vi "initialize python session.vi"(8 "error in (no error)":errorcluster, 11 "Save Image in":refnum<class "Save Image.lvclass">) -> (0 "error out":errorcluster, 3 "Save Image out":refnum<class "Save Image.lvclass">)   [LabVIEW 2018, in "Save Image.lvclass"]
doc: "Initialize the Python Toolkit"
uses:
  Save Image.lvclass
  Save Image.lvclass/Save Image.ctl
  Python Toolkit/Python Toolkit.lvclass/Python Toolkit.ctl
  Python Toolkit/Python Toolkit.lvclass
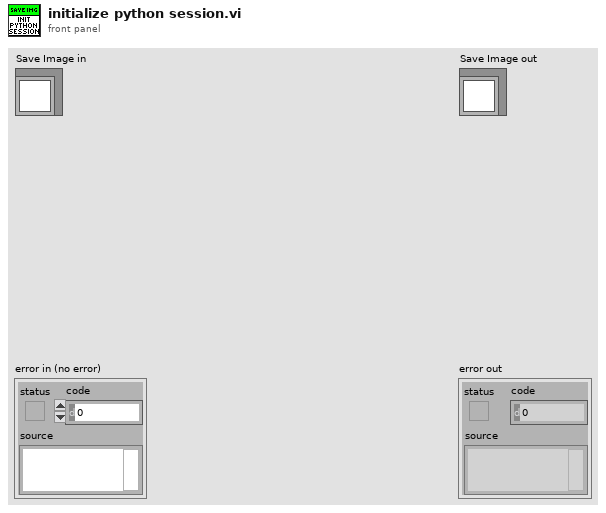
[diagram p1: front panel]
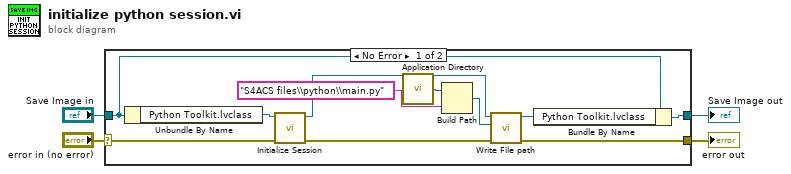
[diagram p0: block diagram]
diagram:
  n1 = case shown="No Error" "error in (no error)" {
    selector: "error in (no error)" -> [w12 w17]
    tunnel: [w9 w17] -> w3
    tunnel: [w14 w16] -> w1
    tunnel: "Save Image in" -> [w13 w16]
    frame No Error {
      n2 = Unbundle By Name(w13) -> ("Python Toolkit.lvclass"=w15:refnum<class "Python Toolkit.lvclass">)
      n3 = call "Initialize Session.vi"("error in (no error)"=w12, "Python Toolkit in"=w15) -> ("error out"=w8:errorcluster, "Python Toolkit out"=w11:refnum<class "Python Toolkit.lvclass">)  [unwired: 8 in]
      n4 = call <vilib>:"Application Directory.vi"() -> ("Application Directory"=w7:path)
      n5 = Build Path(base path=w7, name or relative path="S4ACS files\\python\\main.py") -> (appended path=w5:path)
      n6 = call "Write File path.vi"("error in (no error)"=w8, "File path"=w5, "Python Toolkit in"=w11) -> ("error out"=w9:errorcluster, "Python Toolkit out"=w10:refnum<class "Python Toolkit.lvclass">)  [unwired: 7 in]
      n7 = Bundle By Name(cluster=w13, "Python Toolkit.lvclass"=w10) -> (w14:refnum<class "Save Image.lvclass">)
    }
    frame Error {
    }
  }
  "error out" <- w3
  "Save Image out" <- w1
